vi "StateSpaceUtil_NormalizeInputVector.vi"(7 "J":i32, 9 "Max_Magnitude":dbl, 11 "U":T1) -> (0 "Size Coerced":bool, 3 "NormalizedU":T1)   [LabVIEW 2019, in "Trajectory_Library.lvlib"]
doc: "Normalize all inputs if any excedes the maximum magnitude. Useful for systems such as differential drivetrains.\n \nInputs:\n - J -- The number of inputs.\n - u -- The input vector.\n - maxMagnitude -- The maximum magnitude any input can have.\n\nOutputs:\n - NormalizedU -- The normalizedInput\n - sizeCoerced -- If TRUE, an error occured."
uses:
  Trajectory_Library.lvlib
  <vilib>/Analysis/Matrix/NI_Matrix.lvlib
  <vilib>/Analysis/Matrix/Numeric/Multiply/Multiply - RM,R.vi
  <vilib>/Analysis/Matrix/Datatypes/RealMatrix.ctl
panel:
  # "<J ,1>"
  # "<J ,1>"
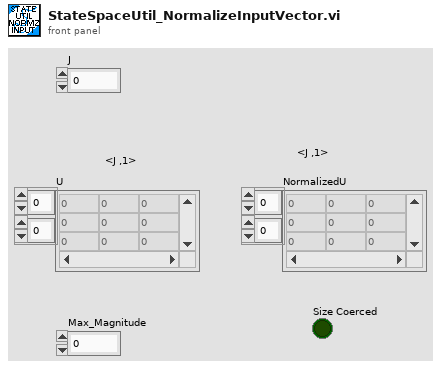
[diagram p1: front panel]
types:
  T1 = typedef "NI_Matrix.lvlib/RealMatrix.ctl" = dbl[][]
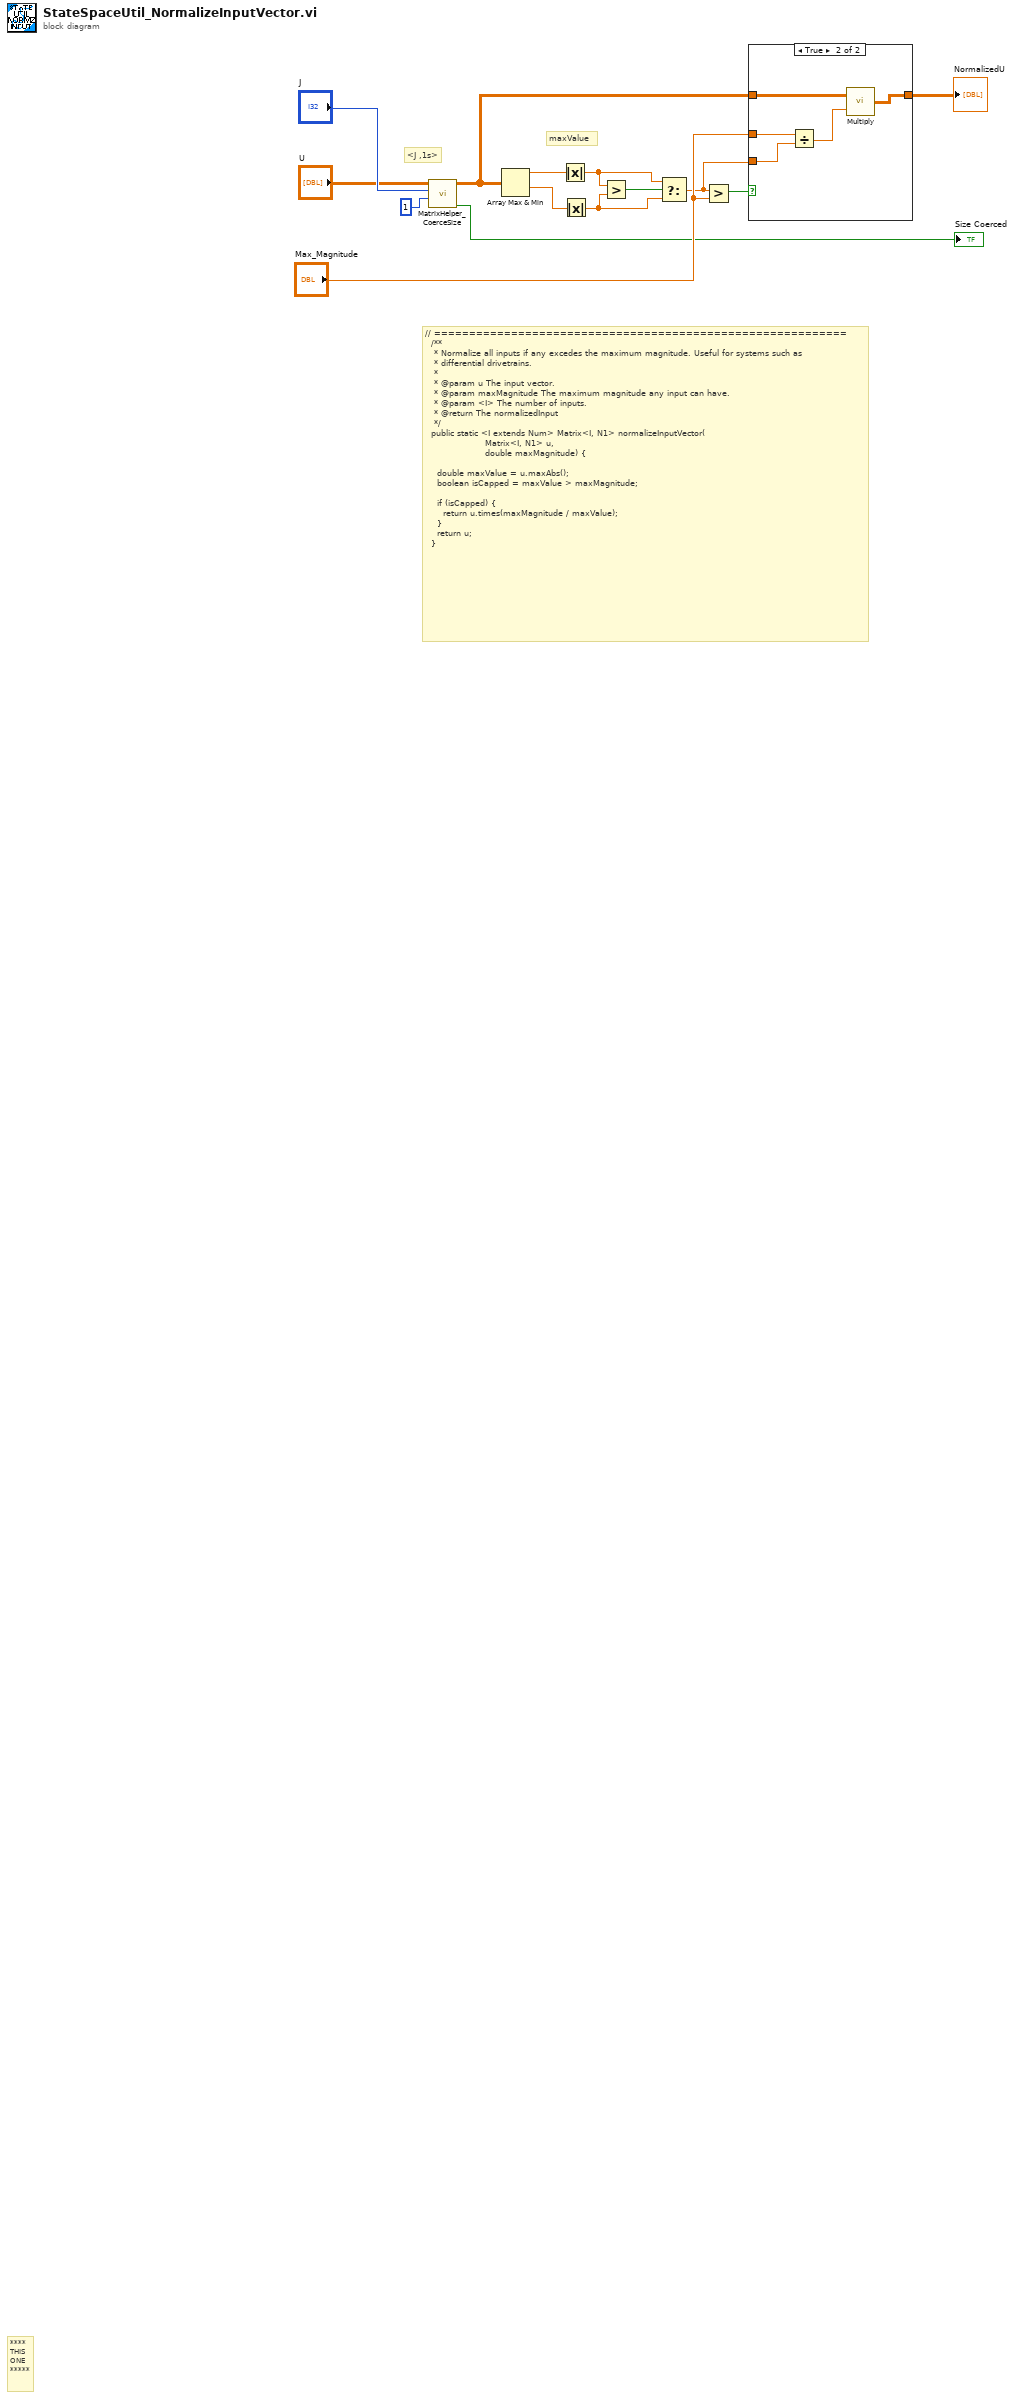
[diagram p0: block diagram]
diagram:
  # "maxValue"
  # "// ===========================================================\n  /**\n   * Normalize all inputs if any excedes the maximum magnitude. Useful for systems such as\n   * differential drivetrains.\n   *\n   * @param u The input vector.\n   * @param maxMagnitude The maximum magnitude any input can have.\n   * @param <I> The number of inputs.\n   * @return The normalizedInput\n   */\n  public static <I extends Num> Matrix<I, N1> normalizeInputVector(\n      \t\t            Matrix<I, N1> u, \n\t        \t          double maxMagnitude) {\n\n    double maxValue = u.maxAbs();\n    boolean isCapped = maxValue > maxMagnitude;\n\n    if (isCapped) {\n      return u.times(maxMagnitude / maxValue);\n    }\n    return u;\n  }"
  # "<J ,1s>"
  # "****\nTHIS\nONE\n*****"
  n1 = call "MatrixHelper_CoerceSize.vi"("Columns"=1 ("number of columns"), "Rows"="J", "input matrix"="U") -> ("Coerced"=→"Size Coerced":bool, "output matrix"=w6:T1)  [unwired: 7 in]
  n2 = Array Max & Min(array=w6) -> (max value=w11:dbl, min value=w10:dbl)  [unwired: 2 out]
  n3 = Absolute Value(x=w11) -> (abs(x)=w9:dbl)
  n4 = Absolute Value(x=w10) -> (abs(x)=w8:dbl)
  n5 = Greater?(x=w9, y=w8) -> (0:w3:bool)
  n6 = Select(t=w9, s=w3, f=w8) -> (s? t:f=w2:dbl)
  n7 = Greater?(x=w2, y="Max_Magnitude") -> (0:w7:bool)
  n8 = case shown="True" w7 {
    tunnel: w6 -> [w15 w18]
    tunnel: [w15 w16] -> w5
    tunnel: "Max_Magnitude" -> [_ w20]
    tunnel: w2 -> [_ w19]
    frame False {
    }
    frame True {
      n9 = Divide(x=w20, y=w19) -> (x/y=w17:dbl)
      n10 = call-poly <vilib>:"Multiply.vi"("Real Scalar c"=w17, "Real Matrix A"=w18) -> ("A * c"=w16:T1)
    }
  }
  "NormalizedU" <- w5
